vi "Error-Ignore.vi"(2 "error in":errorcluster) -> ()   [LabVIEW 2020, in "Sgraph_lib_V1.lvlib"]
doc: "Ignore this error\n\nAndre Koelewijn, sept 2019"
uses:
  Builds/Sgraph_lib_V1.lvlib
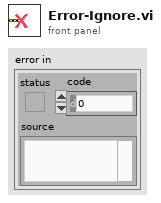
[diagram p1: front panel]
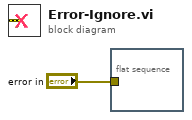
[diagram p0: block diagram]
diagram:
  n1 = flat-sequence {
    tunnel: "error in" -> [_]
    frame #0 {
    }
  }
